vi "Get Message-Enqueuer-References Cluster Reference.vi"(8 "error in (no error)":errorcluster, 11 "VI Refnum in":refnum<vi>) -> (0 "error out":errorcluster, 2 "Cluster":refnum<vi>, 3 "VI Refnum out":refnum<vi>)   [LabVIEW 2018, in "Scripting.lvlib"]
uses:
  Scripting.lvlib
  <vilib>/Utility/traverseref.llb/TRef TravTarget.ctl
  Error-Codes.ctl
  Error-Offset.vi
  <vilib>/Utility/error.llb/Error Cluster From Error Code.vi
  <vilib>/Utility/traverseref.llb/VI Scripting - Traverse.lvlib
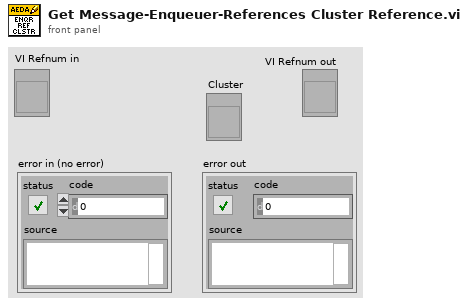
[diagram p1: front panel]
types:
  T1 = typedef "TRef TravTarget.ctl" = enum16{"FP", "BD", "Other"}
  T2 = typedef "Scripting.lvlib/Error-Codes.ctl" = enum16{"EVENT_REF_TYPE_DEF_IS_NESTED", "EVENT_REF_TYPE_DEF_IS_EMPTY", "EVENT_REF_TYPE_DEF_INCLUDES_NON_REFS", "EVENT_REF_TYPE_INVALID_REPLY_REF", "EVENT_REF_TYPE_REPLY_IS_NOT_TYPE_DEF", "EVENT_REF_TYPE_DEF_IS_NOT_CLUSTER", "EVENT_REF_TYPE_DEF_INVALID_REQ_REPLY_TYPE", "ACTOR_CLASS_PATH_IS_INVALID", "ACTOR_CLASS_LIBRARY_IS_NOT_EDITABLE", "ACTOR_CLASS_CREATE_ENQUEUER_REFS_VI_NOT_FOUND", "MSG_ENQUEUER_REFS_CTL_NOT_FOUND", "ACTOR_CLASS_MAIN_RUN_VI_NOT_FOUND", "ACTOR_CLASS_DESTROY_ENQUEUER_REFS_VI_NOT_FOUND", "CREATE_ENQUEUER_REFS_ERROR_TERMINAL_NOT_FOUND", "CREATE_ENQUEUER_REFS_INVALID_TYPE_DEF", "CREATE_ENQUEUER_REF_NAMEBUNDLER_NOT_FOUND", "CREATE_ENQUEUER_REF_MULTIPLE_NAMEBUNDLERS", "MESSAGES_REF_TYPE_DEF_IS_EMPTY", "MESSAGES_REF_TYPE_DEF_IS_NESTED", "ACTOR_TEMPLATE_CLASS_NOT_FOUND"}
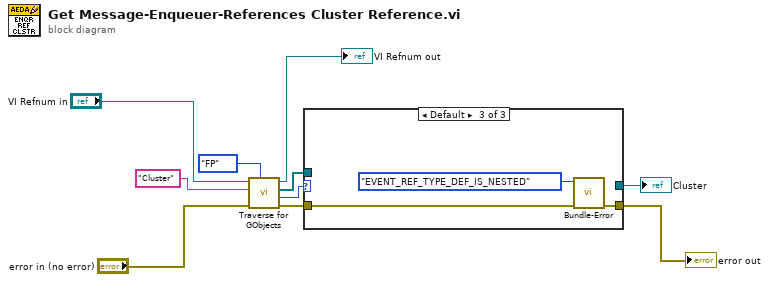
[diagram p0: block diagram]
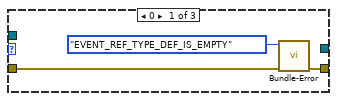
[diagram p2: hidden frame]
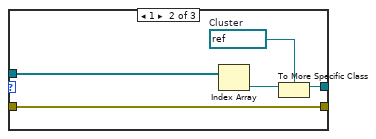
[diagram p3: hidden frame]
diagram:
  n1 = call <vilib>:"Traverse for GObjects.vi"("Traverse Target"=TRef_TravTarget."FP", "error in (no error)"="error in (no error)", "Class Name"="Cluster" ("name/order"), "VI Refnum"="VI Refnum in") -> ("error out"=w6:errorcluster, "# of Refs"=w5:i32, "References"=w8:refnum<vi>[], "dup VI Refnum"=→"VI Refnum out":refnum<vi>)  [unwired: 4 in]
  n2 = case shown="Default" w5 {
    tunnel: w6 -> [w13 w16 w21]
    tunnel: w8 -> [_ w18 _]
    tunnel: [_ w15 _] -> w10
    tunnel: [w11 w16 w19] -> w9
    frame 0 {
      n3 = call "Bundle-Error.vi"("error in (no error)"=w13, "Errors"=Error-Codes."EVENT_REF_TYPE_DEF_IS_EMPTY") -> ("error out"=w11:errorcluster)  [unwired: 9 in]
    }
    frame 1 {
      w14 = refnum<vi> refnum  # Cluster
      n4 = Index Array(array=w18) -> (element=w17:refnum<vi>)  [unwired: 1 in]
      n5 = To More Specific Class(target class=w14, reference=w17) -> (specific class reference=w15:refnum<vi>)  [unwired: 1 in, 1 out]
    }
    frame Default {
      n6 = call "Bundle-Error.vi"("error in (no error)"=w21, "Errors"=Error-Codes."EVENT_REF_TYPE_DEF_IS_NESTED") -> ("error out"=w19:errorcluster)  [unwired: 9 in]
    }
  }
  "Cluster" <- w10
  "error out" <- w9
